vi "AUTOFOCUS_close_calibration_ramp.vi"(0 "queue piezo":refnum<queue>, 1 "z0":dbl, 3 "Ref channel":u16(ring) items=["X signal", "Y signal"], 5 "queue FPGA":refnum<queue>, 7 "Measure QPD":bool, 9 "Channel":bool, 11 "error in":errorcluster, 12 "QPD array":dbl[](array[numeric]), 14 "Z array":dbl[](array[numeric])) -> (4 "Calibration":cluster{"Y":dbl[], "Y":dbl[]}[](graph), 6 "Slope":dbl, 10 "Sensitivity (nm)":dbl, 15 "error out":errorcluster)   [LabVIEW 2015]
uses:
  CONTROLS/Q_MCL_piezo_element.ctl
  CONTROLS/Q_FPGA_element.ctl
  <vilib>/Analysis/NI_AALPro.lvlib
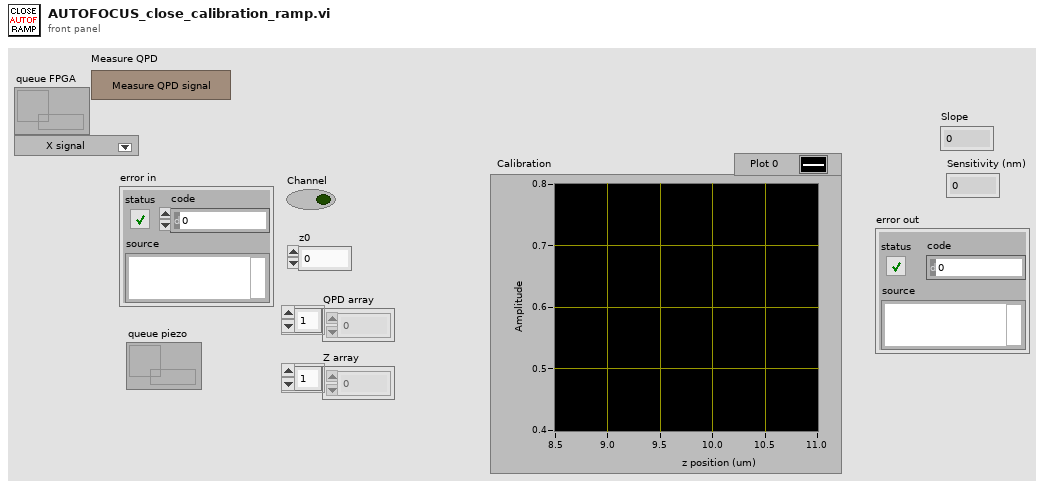
[diagram p1: front panel]
types:
  T1 = typedef "Q_MCL_piezo_element.ctl" = cluster{"variant":variant, "Instruction":enum16{"Piezo_idle", "Piezo_initialize", "Piezo_error", "Piezo_security_stop", "Piezo_read_z", "Piezo_move_z", "Piezo_keyboard_move", "Piezo_close_autofocus_calibration_ramp", "Piezo_change_init_state", "Piezo_init_autofocus", "Piezo_init_autofocus_merFISH_TL", "Piezo_autofocus", "Piezo_autofocus_merFISH_TL", "Piezo_stop_autofocus", "Piezo_stop_autofocus_merFISH_TL", "Piezo_autofocus_lost", "Piezo_resume_autofocus_merFISH_TL", "Piezo_check_z_position_merFISH_TL", "Piezo_init_ramp", "Piezo_move_z_ramp", "Piezo_close_ramp", "Piezo_close_merFISH", "Piezo_stop"}}
  T2 = typedef "Q_FPGA_element.ctl" = cluster{"variant":variant, "Instruction":enum16{"FPGA_idle", "FPGA_initialize", "FPGA_error", "FPGA_security_stop", "FPGA_laser", "FPGA_start_stop_measure_QPD", "FPGA_measure_QPD", "FPGA_measure_QPD_noise", "FPGA_stop_measure_QPD", "FPGA_init_autofocus", "FPGA_init_single_scan", "FPGA_stop_single_scan", "FPGA_init_merFISH", "FPGA_measure_QPD_merFISH", "FPGA_init_scan_merFISH", "FPGA_scan_merFISH", "FPGA_close_merFISH", "FPGA_stop"}}
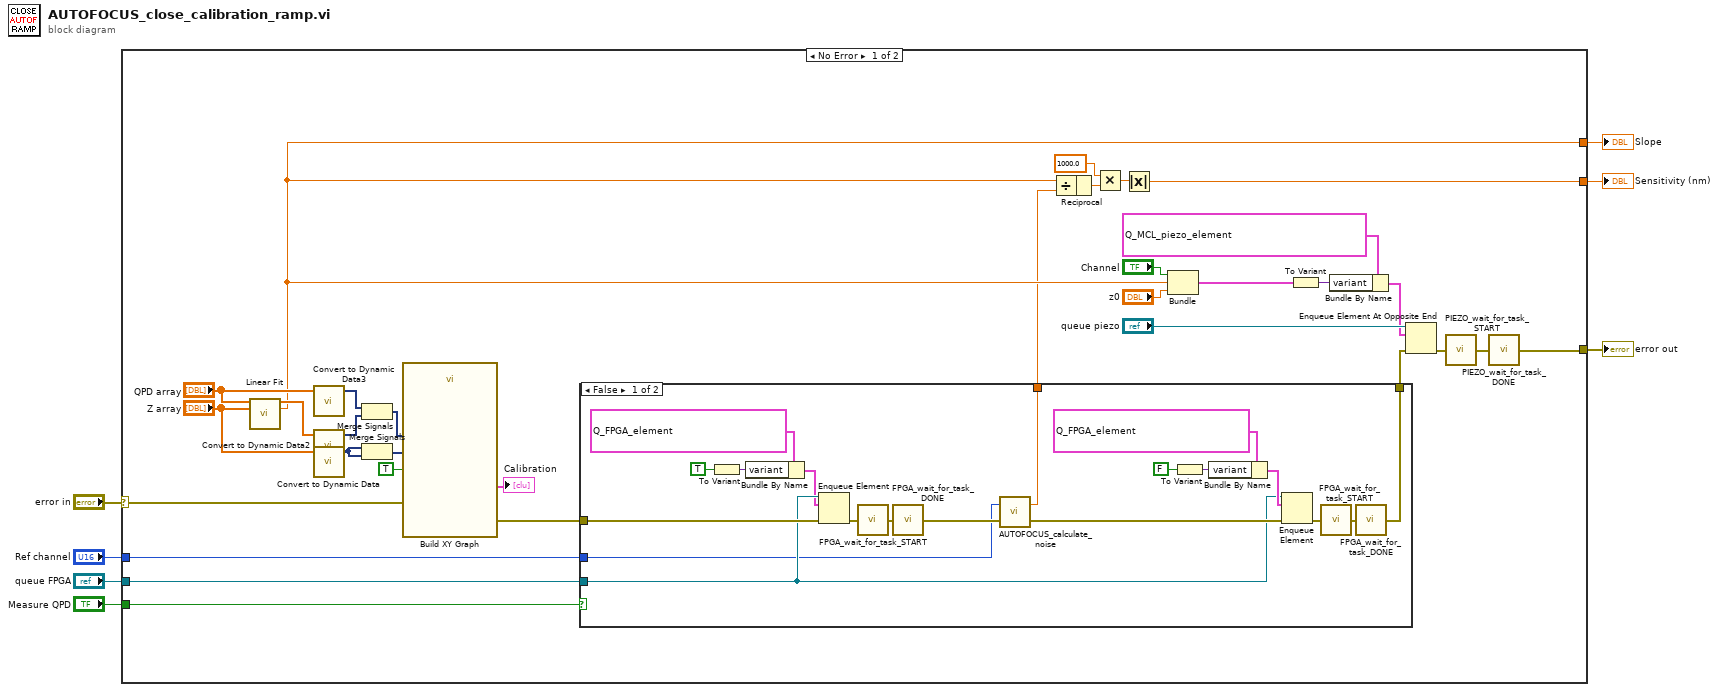
[diagram p0: block diagram]
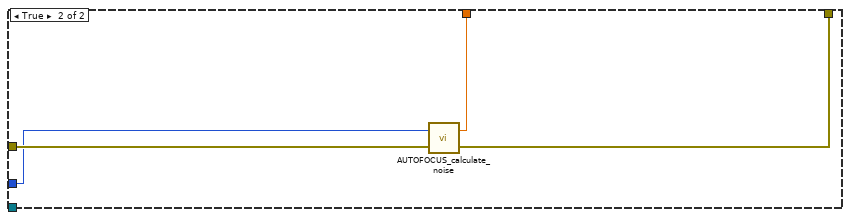
[diagram p2: hidden frame]
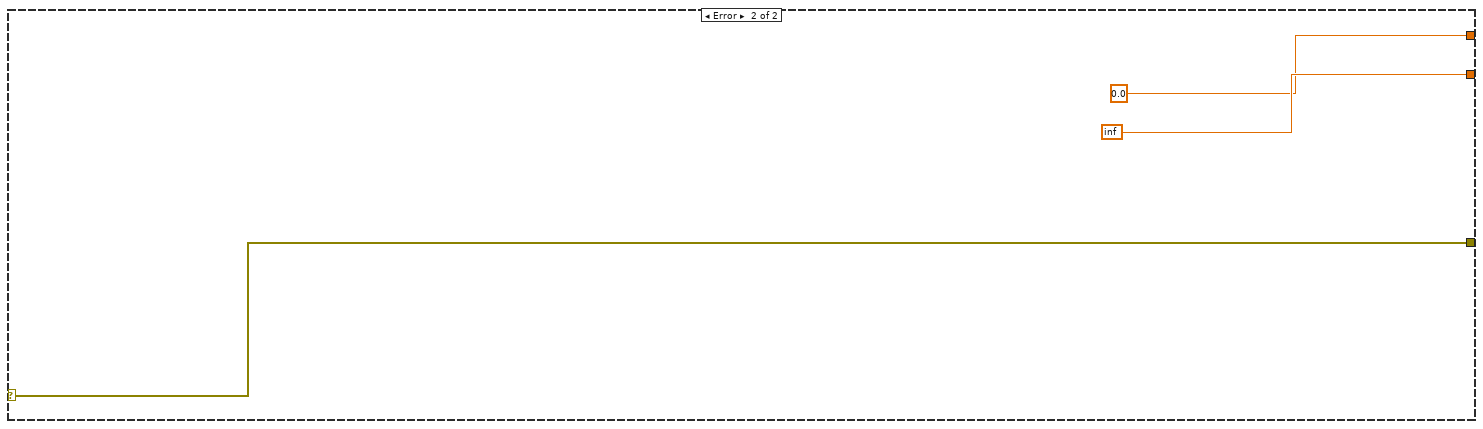
[diagram p3: hidden frame]
diagram:
  n1 = case shown="No Error" "error in" {
    selector: "error in" -> [w25 w66]
    tunnel: [w18 w66] -> w6
    tunnel: [w26 inf] -> w5
    tunnel: [w14 0.0 ("slope")] -> w4
    tunnel: "queue FPGA" -> [w10 _]
    tunnel: "Measure QPD" -> [w9 _]
    tunnel: "Ref channel" -> [w8 _]
    frame No Error {
      n2 = call <vilib>:"Linear Fit.vi"("Y"="QPD array", "X"="Z array") -> ("Best Linear Fit"=w34:dbl[], "slope"=w14:dbl)  [unwired: 9 in, 3 out]
      n3 = call "Convert to Dynamic Data3"("Array"="QPD array") -> ("Dynamic Data Type"=w35:dynamicdata)  [unwired: 3 in]
      n4 = call "Convert to Dynamic Data2"("Array"=w34) -> ("Dynamic Data Type"=w36:dynamicdata)  [unwired: 3 in]
      n5 = call "Convert to Dynamic Data"("Array"="Z array") -> ("Dynamic Data Type"=w39:dynamicdata)  [unwired: 3 in]
      n6 = Merge Signals(w35, w36) -> (w37:dynamicdata)
      n7 = Merge Signals(w39, w39) -> (w38:dynamicdata)
      n8 = call "Build XY Graph"("error in (no error)"=w25, "Reset"=TRUE, "Y Input"=w37, "X Input"=w38) -> ("error out"=w13:errorcluster, "XY Graph"=→"Calibration":cluster{"X":dbl[], "Y":dbl[]}[])  [unwired: 6 in]
      n9 = case shown="False" w9 {
        tunnel: w13 -> [w59 w62]
        tunnel: [w50 w61] -> w12
        tunnel: [w49 w63] -> w11
        tunnel: w10 -> [w48 _]
        tunnel: w8 -> [w41 w60]
        frame False {
          n10 = To Variant(anything=TRUE) -> (Variant=w45:variant)
          n11 = Bundle By Name(cluster=T2 {"variant"=variant, "Instruction"=enum."FPGA_start_stop_measure_QPD"} ("element"), "variant"=w45) -> (w44:T2)
          n12 = Enqueue Element(queue=w48, element=w44, error in (no error)=w59) -> (error out=w47:errorcluster)  [unwired: 1 in, 2 out]
          n13 = call "FPGA_wait_for_task_START.vi"("error in"=w47) -> ("error out"=w46:errorcluster)
          n14 = call "FPGA_wait_for_task_DONE.vi"("error in"=w46) -> ("error out"=w58:errorcluster)
          n15 = call "AUTOFOCUS_calculate_noise.vi"("error in"=w58, "Ref channel"=w41) -> ("error out"=w51:errorcluster, "Noise"=w49:dbl)
          n16 = To Variant(anything=FALSE) -> (Variant=w54:variant)
          n17 = Bundle By Name(cluster=T2 {"variant"=variant, "Instruction"=enum."FPGA_start_stop_measure_QPD"} ("element"), "variant"=w54) -> (w55:T2)
          n18 = Enqueue Element(queue=w48, element=w55, error in (no error)=w51) -> (error out=w52:errorcluster)  [unwired: 1 in, 2 out]
          n19 = call "FPGA_wait_for_task_START.vi"("error in"=w52) -> ("error out"=w53:errorcluster)
          n20 = call "FPGA_wait_for_task_DONE.vi"("error in"=w53) -> ("error out"=w50:errorcluster)
        }
        frame True {
          n21 = call "AUTOFOCUS_calculate_noise.vi"("error in"=w62, "Ref channel"=w60) -> ("error out"=w61:errorcluster, "Noise"=w63:dbl)
        }
      }
      n22 = Divide(x=w14, y=w11) -> (x/y=w27:dbl)
      n23 = Reciprocal(x=w27) -> (1/x=w30:dbl)
      n24 = Multiply(x=1000.0, y=w30) -> (x*y=w29:dbl)
      n25 = Absolute Value(x=w29) -> (abs(x)=w26:dbl)
      n26 = Bundle("Channel"="Channel", "slope"=w14, "z0"="z0") -> (w16:cluster{"Channel":bool, "slope":dbl, "z0":dbl})  [unwired: 1 in]
      n27 = To Variant(anything=w16) -> (Variant=w22:variant)
      n28 = Bundle By Name(cluster=T1 {"variant"=variant, "Instruction"=enum."Piezo_close_autofocus_calibration_ramp"} ("element"), "variant"=w22) -> (w21:T1)
      n29 = Enqueue Element At Opposite End(queue="queue piezo", element=w21, error in (no error)=w12) -> (error out=w20:errorcluster)  [unwired: 1 in, 2 out]
      n30 = call "PIEZO_wait_for_task_START.vi"("error in"=w20) -> ("error out"=w19:errorcluster)
      n31 = call "PIEZO_wait_for_task_DONE.vi"("error in"=w19) -> ("error out"=w18:errorcluster)
    }
    frame Error {
    }
  }
  "error out" <- w6
  "Sensitivity (nm)" <- w5
  "Slope" <- w4
